vi "Msg To Self.vi"(9 "Priority?":bool, 10 "Msg":refnum<class "Msg.lvclass">, 11 "Dev Actor in":refnum<class "Dev Actor.lvclass">) -> (0 "error out":errorcluster)   [LabVIEW 2021, in "Dev Actor.lvlib" / "Dev Actor.lvclass"]
uses:
  Dev Actor.lvclass
  Actor/Msg/Msg.lvclass
  Dev Actor.lvclass/Dev Actor.ctl
  Queue Actor/Queue Actor.lvclass
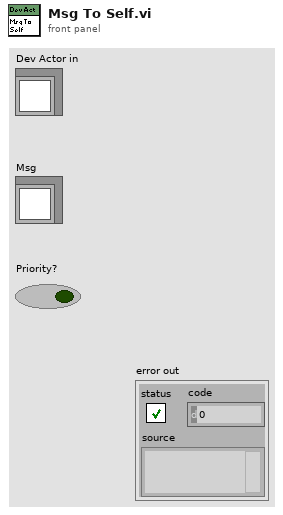
[diagram p1: front panel]
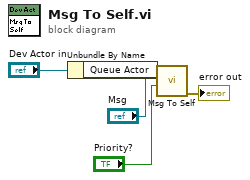
[diagram p0: block diagram]
diagram:
  n1 = Unbundle By Name("Dev Actor in") -> ("Queue Actor"=w4:refnum<class "Queue Actor.lvclass">)
  n2 = call-dynamic "Msg To Self.vi"("Priority?"="Priority?", "Msg"="Msg", "Queue Actor in"=w4) -> ("error out"=→"error out":errorcluster)  [unwired: 8 in]
